vi "Git-Get Repositories.vi"() -> ()   [LabVIEW 2020]
uses:
  Git-Repo JSON Typedef.ctl
  <vilib>/addons/_JKI.lib/REST Client/classes/REST Client/REST Client.lvclass
  <vilib>/JDP Science/JSONtext/JSONtext.lvlib
panel:
  out "Array":T1[](array[typedef])
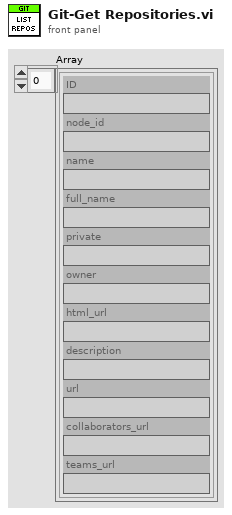
[diagram p1: front panel]
types:
  T1 = typedef "Git-Repo JSON Typedef.ctl" = cluster{"ID":string, "node_id":string, "name":string, "full_name":string, "private":string, "owner":string, "html_url":string, "description":string, "url":string, "collaborators_url":string, "teams_url":string}
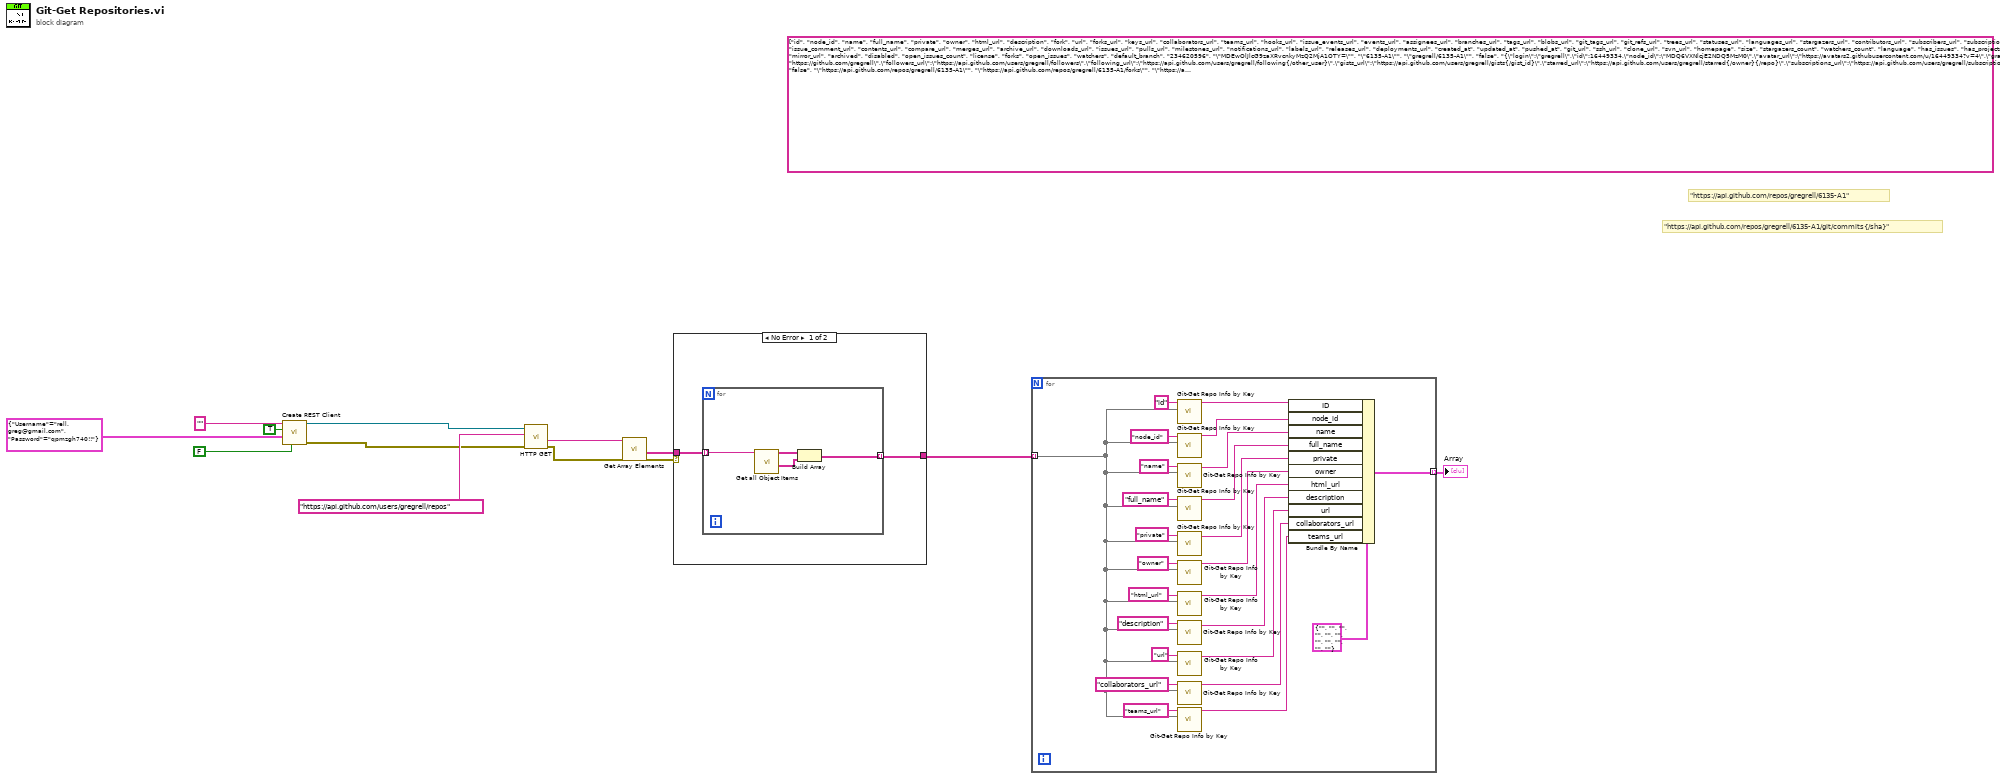
[diagram p0: block diagram]
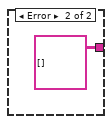
[diagram p2: hidden frame]
diagram:
  (unwired) string[][][] [[["id", "node_id", "name", "full_name", "private", "owner", "html_url", "description", "fork", "url", "forks_url", "keys_url", "collaborators_url", "teams_url", "hooks_url", "issue_events_url", "events_url", "assignees_url", "branches_url", "tags_url", "blobs_url", "git_tags_url", "git_refs_url", "trees_url", "statuses_url", "languages_url", "stargazers_url", "contributors_url", "subscribers_url", "subscription_url", "commits_url", "git_commits_url", "comments_url", "issue_comment_url", "contents_url", "compare_url", "merges_url", "archive_url", "downloads_url", "issues_url", "pulls_url", "milestones_url", "notifications_url", "labels_url", "releases_url", "deployments_url", "created_at", "updated_at", "pushed_at", "git_url", "ssh_url", "clone_url", "svn_url", "homepage", "size", "stargazers_count", "watchers_count", "language", "has_issues", "has_projects", "has_downloads", "has_wiki", "has_pages", "forks_count", "mirror_url", "archived", "disabled", "open_issues_count", "license", "forks", "open_issues", "watchers", "default_branch"], ["234620596", "\"MDEwOlJlcG9zaXRvcnkyMzQ2MjA1OTY=\"", "\"6135-A1\"", "\"gregrell/6135-A1\"", "false", "{\"login\":\"gregrell\",\"id\":16449334,\"node_id\":\"MDQ6VXNlcjE2NDQ5MzM0\",\"avatar_url\":\"https://avatars2.githubusercontent.com/u/16449334?v=4\",\"gravatar_id\":\"\",\"url\":\"https://api.github.com/users/gregrell\",\"html_url\":\"https://github.com/gregrell\",\"followers_url\":\"https://api.github.com/users/gregrell/followers\",\"following_url\":\"https://api.github.com/users/gregrell/following{/other_user}\",\"gists_url\":\"https://api.github.com/users/gregrell/gists{/gist_id}\",\"starred_url\":\"https://api.github.com/users/gregrell/starred{/owner}{/repo}\",\"subscriptions_url\":\"https://api.github.com/users/gregrell/subscriptions\",\"organizations_url\":\"https://api.github.com/users/gregrell/orgs\",\"repos_url\":\"https://api.github.com/users/gregrell/repos\",\"events_url\":\"https://api.github.com/users/gregrell/events{/privacy}\",\"received_events_url\":\"https://api.github.com/users/gregrell/received_events\",\"type\":\"User\",\"site_admin\":false}", "\"https://github.com/gregrell/6135-A1\"", "\"Assignment 1\"", "false", "\"https://api.github.com/repos/gregrell/6135-A1\"", "\"https://api.github.com/repos/gregrell/6135-A1/forks\"", "\"https://api.github.com/repos/gregrell/6135-A1/keys{/key_id}\"", "\"https://api.github.com/repos/gregrell/6135-A1/collaborators{/collaborator}\"", "\"https://api.github.com/repos/gregrell/6135-A1/teams\"", "\"https://api.github.com/repos/gregrell/6135-A1/hooks\"", "\"https://api.github.com/repos/gregrell/6135-A1/issues/events{/number}\"", "\"https://api.github.com/repos/gregrell/6135-A1/events\"", "\"https://api.github.com/repos/gregrell/6135-A1/assignees{/user}\"", "\"https://api.github.com/repos/gregrell/6135-A1/branches{/branch}\"", "\"https://api.github.com/repos/gregrell/6135-A1/tags\"", "\"https://api.github.com/repos/gregrell/6135-A1/git/blobs{/sha}\"", "\"https://api.github.com/repos/gregrell/6135-A1/git/tags{/sha}\"", "\"https://api.github.com/repos/gregrell/6135-A1/git/refs{/sha}\"", "\"https://api.github.com/repos/gregrell/6135-A1/git/trees{/sha}\"", "\"https://api.github.com/repos/gregrell/6135-A1/statuses/{sha}\"", "\"https://api.github.com/repos/gregrell/6135-A1/languages\"", "\"https://api.github.com/repos/gregrell/6135-A1/stargazers\"", "\"https://api.github.com/repos/gregrell/6135-A1/contributors\"", "\"https://api.github.com/repos/gregrell/6135-A1/subscribers\"", "\"https://api.github.com/repos/gregrell/6135-A1/subscription\"", "\"https://api.github.com/repos/gregrell/6135-A1/commits{/sha}\"", "\"https://api.github.com/repos/gregrell/6135-A1/git/commits{/sha}\"", "\"https://api.github.com/repos/gregrell/6135-A1/comments{/number}\"", "\"https://api.github.com/repos/gregrell/6135-A1/issues/comments{/number}\"", "\"https://api.github.com/repos/gregrell/6135-A1/contents/{+path}\"", "\"https://api.github.com/repos/gregrell/6135-A1/compare/{base}...{head}\"", "\"https://api.github.com/repos/gregrell/6135-A1/merges\"", "\"https://api.github.com/repos/gregrell/6135-A1/{archive_format}{/ref}\"", "\"https://api.github.com/repos/gregrell/6135-A1/downloads\"", "\"https://api.github.com/repos/gregrell/6135-A1/issues{/number}\"", "\"https://api.github.com/repos/gregrell/6135-A1/pulls{/number}\"", "\"https://api.github.com/repos/gregrell/6135-A1/milestones{/number}\"", "\"https://api.github.com/repos/gregrell/6135-A1/notifications{?since,all,participating}\"", "\"https://api.github.com/repos/gregrell/6135-A1/labels{/name}\"", "\"https://api.github.com/repos/gregrell/6135-A1/releases{/id}\"", "\"https://api.github.com/repos/gregrell/6135-A1/deployments\"", "\"2020-01-17T19:21:34Z\"", "\"2020-02-04T17:49:57Z\"", "\"2020-02-04T17:49:55Z\"", "\"git://github.com/gregrell/6135-A1.git\"", "\"git@github.com:gregrell/6135-A1.git\"", "\"https://github.com/gregrell/6135-A1.git\"", "\"https://github.com/gregrell/6135-A1\"", "null", "12", "0", "0", "\"C\"", "true", "true", "true", "true", "false", "0", "null", "false", "false", "0", "null", "0", "0", "0", "\"master\""]], [["id", "node_id", "name", "full_name", "private", "owner", "html_url", "description", "fork", "url", "forks_url", "keys_url", "collaborators_url", "teams_url", "hooks_url", "issue_events_url", "events_url", "assignees_url", "branches_url", "tags_url", "blobs_url", "git_tags_url", "git_refs_url", "trees_url", "statuses_url", "languages_url", "stargazers_url", "contributors_url", "subscribers_url", "subscription_url", "commits_url", "git_commits_url", "comments_url", "issue_comment_url", "contents_url", "compare_url", "merges_url", "archive_url", "downloads_url", "issues_url", "pulls_url", "milestones_url", "notifications_url", "labels_url", "releases_url", "deployments_url", "created_at", "updated_at", "pushed_at", "git_url", "ssh_url", "clone_url", "svn_url", "homepage", "size", "stargazers_count", "watchers_count", "language", "has_issues", "has_projects", "has_downloads", "has_wiki", "has_pages", "forks_count", "mirror_url", "archived", "disabled", "open_issues_count", "license", "forks", "open_issues", "watchers", "default_branch"], ["244166740", "\"MDEwOlJlcG9zaXRvcnkyNDQxNjY3NDA=\"", "\"6135-A2\"", "\"gregrell/6135-A2\"", "false", "{\"login\":\"gregrell\",\"id\":16449334,\"node_id\":\"MDQ6VXNlcjE2NDQ5MzM0\",\"avatar_url\":\"https://avatars2.githubusercontent.com/u/16449334?v=4\",\"gravatar_id\":\"\",\"url\":\"https://api.github.com/users/gregrell\",\"html_url\":\"https://github.com/gregrell\",\"followers_url\":\"https://api.github.com/users/gregrell/followers\",\"following_url\":\"https://api.github.com/users/gregrell/following{/other_user}\",\"gists_url\":\"https://api.github.com/users/gregrell/gists{/gist_id}\",\"starred_url\":\"https://api.github.com/users/gregrell/starred{/owner}{/repo}\",\"subscriptions_url\":\"https://api.github.com/users/gregrell/subscriptions\",\"organizations_url\":\"https://api.github.com/users/gregrell/orgs\",\"repos_url\":\"https://api.github.com/users/gregrell/repos\",\"events_url\":\"https://api.github.com/users/gregrell/events{/privacy}\",\"received_events_url\":\"https://api.github.com/users/gregrell/received_events\",\"type\":\"User\",\"site_admin\":false}", "\"https://github.com/gregrell/6135-A2\"", "null", "false", "\"https://api.github.com/repos/gregrell/6135-A2\"", "\"https://api.github.com/repos/gregrell/6135-A2/forks\"", "\"https://api.github.com/repos/gregrell/6135-A2/keys{/key_id}\"", "\"https://api.github.com/repos/gregrell/6135-A2/collaborators{/collaborator}\"", "\"https://api.github.com/repos/gregrell/6135-A2/teams\"", "\"https://api.github.com/repos/gregrell/6135-A2/hooks\"", "\"https://api.github.com/repos/gregrell/6135-A2/issues/events{/number}\"", "\"https://api.github.com/repos/gregrell/6135-A2/events\"", "\"https://api.github.com/repos/gregrell/6135-A2/assignees{/user}\"", "\"https://api.github.com/repos/gregrell/6135-A2/branches{/branch}\"", "\"https://api.github.com/repos/gregrell/6135-A2/tags\"", "\"https://api.github.com/repos/gregrell/6135-A2/git/blobs{/sha}\"", "\"https://api.github.com/repos/gregrell/6135-A2/git/tags{/sha}\"", "\"https://api.github.com/repos/gregrell/6135-A2/git/refs{/sha}\"", "\"https://api.github.com/repos/gregrell/6135-A2/git/trees{/sha}\"", "\"https://api.github.com/repos/gregrell/6135-A2/statuses/{sha}\"", "\"https://api.github.com/repos/gregrell/6135-A2/languages\"", "\"https://api.github.com/repos/gregrell/6135-A2/stargazers\"", "\"https://api.github.com/repos/gregrell/6135-A2/contributors\"", "\"https://api.github.com/repos/gregrell/6135-A2/subscribers\"", "\"https://api.github.com/repos/gregrell/6135-A2/subscription\"", "\"https://api.github.com/repos/gregrell/6135-A2/commits{/sha}\"", "\"https://api.github.com/repos/gregrell/6135-A2/git/commits{/sha}\"", "\"https://api.github.com/repos/gregrell/6135-A2/comments{/number}\"", "\"https://api.github.com/repos/gregrell/6135-A2/issues/comments{/number}\"", "\"https://api.github.com/repos/gregrell/6135-A2/contents/{+path}\"", "\"https://api.github.com/repos/gregrell/6135-A2/compare/{base}...{head}\"", "\"https://api.github.com/repos/gregrell/6135-A2/merges\"", "\"https://api.github.com/repos/gregrell/6135-A2/{archive_format}{/ref}\"", "\"https://api.github.com/repos/gregrell/6135-A2/downloads\"", "\"https://api.github.com/repos/gregrell/6135-A2/issues{/number}\"", "\"https://api.github.com/repos/gregrell/6135-A2/pulls{/number}\"", "\"https://api.github.com/repos/gregrell/6135-A2/milestones{/number}\"", "\"https://api.github.com/repos/gregrell/6135-A2/notifications{?since,all,participating}\"", "\"https://api.github.com/repos/gregrell/6135-A2/labels{/name}\"", "\"https://api.github.com/repos/gregrell/6135-A2/releases{/id}\"", "\"https://api.github.com/repos/gregrell/6135-A2/deployments\"", "\"2020-03-01T14:45:42Z\"", "\"2020-03-03T01:29:14Z\"", "\"2020-03-03T01:29:12Z\"", "\"git://github.com/gregrell/6135-A2.git\"", "\"git@github.com:gregrell/6135-A2.git\"", "\"https://github.com/gregrell/6135-A2.git\"", "\"https://github.com/gregrell/6135-A2\"", "null", "3", "0", "0", "\"Python\"", "true", "true", "true", "true", "false", "0", "null", "false", "false", "1", "null", "0", "1", "0", "\"master\""]], [["id", "node_id", "name", "full_name", "private", "owner", "html_url", "description", "fork", "url", "forks_url", "keys_url", "collaborators_url", "teams_url", "hooks_url", "issue_events_url", "events_url", "assignees_url", "branches_url", "tags_url", "blobs_url", "git_tags_url", "git_refs_url", "trees_url", "statuses_url", "languages_url", "stargazers_url", "contributors_url", "subscribers_url", "subscription_url", "commits_url", "git_commits_url", "comments_url", "issue_comment_url", "contents_url", "compare_url", "merges_url", "archive_url", "downloads_url", "issues_url", "pulls_url", "milestones_url", "notifications_url", "labels_url", "releases_url", "deployments_url", "created_at", "updated_at", "pushed_at", "git_url", "ssh_url", "clone_url", "svn_url", "homepage", "size", "stargazers_count", "watchers_count", "language", "has_issues", "has_projects", "has_downloads", "has_wiki", "has_pages", "forks_count", "mirror_url", "archived", "disabled", "open_issues_count", "license", "forks", "open_issues", "watchers", "default_branch"], ["102971263", "\"MDEwOlJlcG9zaXRvcnkxMDI5NzEyNjM=\"", "\"AIPacMan1\"", "\"gregrell/AIPacMan1\"", "false", "{\"login\":\"gregrell\",\"id\":16449334,\"node_id\":\"MDQ6VXNlcjE2NDQ5MzM0\",\"avatar_url\":\"https://avatars2.githubusercontent.com/u/16449334?v=4\",\"gravatar_id\":\"\",\"url\":\"https://api.github.com/users/gregrell\",\"html_url\":\"https://github.com/gregrell\",\"followers_url\":\"https://api.github.com/users/gregrell/followers\",\"following_url\":\"https://api.github.com/users/gregrell/following{/other_user}\",\"gists_url\":\"https://api.github.com/users/gregrell/gists{/gist_id}\",\"starred_url\":\"https://api.github.com/users/gregrell/starred{/owner}{/repo}\",\"subscriptions_url\":\"https://api.github.com/users/gregrell/subscriptions\",\"organizations_url\":\"https://api.github.com/users/gregrell/orgs\",\"repos_url\":\"https://api.github.com/users/gregrell/repos\",\"events_url\":\"https://api.github.com/users/gregrell/events{/privacy}\",\"received_events_url\":\"https://api.github.com/users/gregrell/received_events\",\"type\":\"User\",\"site_admin\":false}", "\"https://github.com/gregrell/AIPacMan1\"", "\"AI Class Pacman assignment 1\"", "false", "\"https://api.github.com/repos/gregrell/AIPacMan1\"", "\"https://api.github.com/repos/gregrell/AIPacMan1/forks\"", "\"https://api.github.com/repos/gregrell/AIPacMan1/keys{/key_id}\"", "\"https://api.github.com/repos/gregrell/AIPacMan1/collaborators{/collaborator}\"", "\"https://api.github.com/repos/gregrell/AIPacMan1/teams\"", "\"https://api.github.com/repos/gregrell/AIPacMan1/hooks\"", "\"https://api.github.com/repos/gregrell/AIPacMan1/issues/events{/number}\"", "\"https://api.github.com/repos/gregrell/AIPacMan1/events\"", "\"https://api.github.com/repos/gregrell/AIPacMan1/assignees{/user}\"", "\"https://api.github.com/repos/gregrell/AIPacMan1/branches{/branch}\"", "\"https://api.github.com/repos/gregrell/AIPacMan1/tags\"", "\"https://api.github.com/repos/gregrell/AIPacMan1/git/blobs{/sha}\"", "\"https://api.github.com/repos/gregrell/AIPacMan1/git/tags{/sha}\"", "\"https://api.github.com/repos/gregrell/AIPacMan1/git/refs{/sha}\"", "\"https://api.github.com/repos/gregrell/AIPacMan1/git/trees{/sha}\"", "\"https://api.github.com/repos/gregrell/AIPacMan1/statuses/{sha}\"", "\"https://api.github.com/repos/gregrell/AIPacMan1/languages\"", "\"https://api.github.com/repos/gregrell/AIPacMan1/stargazers\"", "\"https://api.github.com/repos/gregrell/AIPacMan1/contributors\"", "\"https://api.github.com/repos/gregrell/AIPacMan1/subscribers\"", "\"https://api.github.com/repos/gregrell/AIPacMan1/subscription\"", "\"https://api.github.com/repos/gregrell/AIPacMan1/commits{/sha}\"", "\"https://api.github.com/repos/gregrell/AIPacMan1/git/commits{/sha}\"", "\"https://api.github.com/repos/gregrell/AIPacMan1/comments{/number}\"", "\"https://api.github.com/repos/gregrell/AIPacMan1/issues/comments{/number}\"", "\"https://api.github.com/repos/gregrell/AIPacMan1/contents/{+path}\"", "\"https://api.github.com/repos/gregrell/AIPacMan1/compare/{base}...{head}\"", "\"https://api.github.com/repos/gregrell/AIPacMan1/merges\"", "\"https://api.github.com/repos/gregrell/AIPacMan1/{archive_format}{/ref}\"", "\"https://api.github.com/repos/gregrell/AIPacMan1/downloads\"", "\"https://api.github.com/repos/gregrell/AIPacMan1/issues{/number}\"", "\"https://api.github.com/repos/gregrell/AIPacMan1/pulls{/number}\"", "\"https://api.github.com/repos/gregrell/AIPacMan1/milestones{/number}\"", "\"https://api.github.com/repos/gregrell/AIPacMan1/notifications{?since,all,participating}\"", "\"https://api.github.com/repos/gregrell/AIPacMan1/labels{/name}\"", "\"https://api.github.com/repos/gregrell/AIPacMan1/releases{/id}\"", "\"https://api.github.com/repos/gregrell/AIPacMan1/deployments\"", "\"2017-09-09T17:04:38Z\"", "\"2017-09-09T17:06:54Z\"", "\"2017-10-05T17:59:55Z\"", "\"git://github.com/gregrell/AIPacMan1.git\"", "\"git@github.com:gregrell/AIPacMan1.git\"", "\"https://github.com/gregrell/AIPacMan1.git\"", "\"https://github.com/gregrell/AIPacMan1\"", "null", "277", "0", "0", "\"Python\"", "true", "true", "true", "true", "false", "0", "null", "false", "false", "0", "null", "0", "0", "0", "\"master\""]], [["id", "node_id", "name", "full_name", "private", "owner", "html_url", "description", "fork", "url", "forks_url", "keys_url", "collaborators_url", "teams_url", "hooks_url", "issue_events_url", "events_url", "assignees_url", "branches_url", "tags_url", "blobs_url", "git_tags_url", "git_refs_url", "trees_url", "statuses_url", "languages_url", "stargazers_url", "contributors_url", "subscribers_url", "subscription_url", "commits_url", "git_commits_url", "comments_url", "issue_comment_url", "contents_url", "compare_url", "merges_url", "archive_url", "downloads_url", "issues_url", "pulls_url", "milestones_url", "notifications_url", "labels_url", "releases_url", "deployments_url", "created_at", "updated_at", "pushed_at", "git_url", "ssh_url", "clone_url", "svn_url", "homepage", "size", "stargazers_count", "watchers_count", "language", "has_issues", "has_projects", "has_downloads", "has_wiki", "has_pages", "forks_count", "mirror_url", "archived", "disabled", "open_issues_count", "license", "forks", "open_issues", "watchers", "default_branch"], ["108994983", "\"MDEwOlJlcG9zaXRvcnkxMDg5OTQ5ODM=\"", "\"AIPacMan2\"", "\"gregrell/AIPacMan2\"", "false", "{\"login\":\"gregrell\",\"id\":16449334,\"node_id\":\"MDQ6VXNlcjE2NDQ5MzM0\",\"avatar_url\":\"https://avatars2.githubusercontent.com/u/16449334?v=4\",\"gravatar_id\":\"\",\"url\":\"https://api.github.com/users/gregrell\",\"html_url\":\"https://github.com/gregrell\",\"followers_url\":\"https://api.github.com/users/gregrell/followers\",\"following_url\":\"https://api.github.com/users/gregrell/following{/other_user}\",\"gists_url\":\"https://api.github.com/users/gregrell/gists{/gist_id}\",\"starred_url\":\"https://api.github.com/users/gregrell/starred{/owner}{/repo}\",\"subscriptions_url\":\"https://api.github.com/users/gregrell/subscriptions\",\"organizations_url\":\"https://api.github.com/users/gregrell/orgs\",\"repos_url\":\"https://api.github.com/users/gregrell/repos\",\"events_url\":\"https://api.github.com/users/gregrell/events{/privacy}\",\"received_events_url\":\"https://api.github.com/users/gregrell/received_events\",\"type\":\"User\",\"site_admin\":false}", "\"https://github.com/gregrell/AIPacMan2\"", "\"Berkley AI course project 3\"", "false", "\"https://api.github.com/repos/gregrell/AIPacMan2\"", "\"https://api.github.com/repos/gregrell/AIPacMan2/forks\"", "\"https://api.github.com/repos/gregrell/AIPacMan2/keys{/key_id}\"", "\"https://api.github.com/repos/gregrell/AIPacMan2/collaborators{/collaborator}\"", "\"https://api.github.com/repos/gregrell/AIPacMan2/teams\"", "\"https://api.github.com/repos/gregrell/AIPacMan2/hooks\"", "\"https://api.github.com/repos/gregrell/AIPacMan2/issues/events{/number}\"", "\"https://api.github.com/repos/gregrell/AIPacMan2/events\"", "\"https://api.github.com/repos/gregrell/AIPacMan2/assignees{/user}\"", "\"https://api.github.com/repos/gregrell/AIPacMan2/branches{/branch}\"", "\"https://api.github.com/repos/gregrell/AIPacMan2/tags\"", "\"https://api.github.com/repos/gregrell/AIPacMan2/git/blobs{/sha}\"", "\"https://api.github.com/repos/gregrell/AIPacMan2/git/tags{/sha}\"", "\"https://api.github.com/repos/gregrell/AIPacMan2/git/refs{/sha}\"", "\"https://api.github.com/repos/gregrell/AIPacMan2/git/trees{/sha}\"", "\"https://api.github.com/repos/gregrell/AIPacMan2/statuses/{sha}\"", "\"https://api.github.com/repos/gregrell/AIPacMan2/languages\"", "\"https://api.github.com/repos/gregrell/AIPacMan2/stargazers\"", "\"https://api.github.com/repos/gregrell/AIPacMan2/contributors\"", "\"https://api.github.com/repos/gregrell/AIPacMan2/subscribers\"", "\"https://api.github.com/repos/gregrell/AIPacMan2/subscription\"", "\"https://api.github.com/repos/gregrell/AIPacMan2/commits{/sha}\"", "\"https://api.github.com/repos/gregrell/AIPacMan2/git/commits{/sha}\"", "\"https://api.github.com/repos/gregrell/AIPacMan2/comments{/number}\"", "\"https://api.github.com/repos/gregrell/AIPacMan2/issues/comments{/number}\"", "\"https://api.github.com/repos/gregrell/AIPacMan2/contents/{+path}\"", "\"https://api.github.com/repos/gregrell/AIPacMan2/compare/{base}...{head}\"", "\"https://api.github.com/repos/gregrell/AIPacMan2/merges\"", "\"https://api.github.com/repos/gregrell/AIPacMan2/{archive_format}{/ref}\"", "\"https://api.github.com/repos/gregrell/AIPacMan2/downloads\"", "\"https://api.github.com/repos/gregrell/AIPacMan2/issues{/number}\"", "\"https://api.github.com/repos/gregrell/AIPacMan2/pulls{/number}\"", "\"https://api.github.com/repos/gregrell/AIPacMan2/milestones{/number}\"", "\"https://api.github.com/repos/gregrell/AIPacMan2/notifications{?since,all,participating}\"", "\"https://api.github.com/repos/gregrell/AIPacMan2/labels{/name}\"", "\"https://api.github.com/repos/gregrell/AIPacMan2/releases{/id}\"", "\"https://api.github.com/repos/gregrell/AIPacMan2/deployments\"", "\"2017-10-31T12:50:33Z\"", "\"2017-10-31T12:54:09Z\"", "\"2017-11-19T15:26:08Z\"", "\"git://github.com/gregrell/AIPacMan2.git\"", "\"git@github.com:gregrell/AIPacMan2.git\"", "\"https://github.com/gregrell/AIPacMan2.git\"", "\"https://github.com/gregrell/AIPacMan2\"", "null", "421", "0", "0", "\"Python\"", "true", "true", "true", "true", "false", "0", "null", "false", "false", "0", "null", "0", "0", "0", "\"master\""]], [["id", "node_id", "name", "full_name", "private", "owner", "html_url", "description", "fork", "url", "forks_url", "keys_url", "collaborators_url", "teams_url", "hooks_url", "issue_events_url", "events_url", "assignees_url", "branches_url", "tags_url", "blobs_url", "git_tags_url", "git_refs_url", "trees_url", "statuses_url", "languages_url", "stargazers_url", "contributors_url", "subscribers_url", "subscription_url", "commits_url", "git_commits_url", "comments_url", "issue_comment_url", "contents_url", "compare_url", "merges_url", "archive_url", "downloads_url", "issues_url", "pulls_url", "milestones_url", "notifications_url", "labels_url", "releases_url", "deployments_url", "created_at", "updated_at", "pushed_at", "git_url", "ssh_url", "clone_url", "svn_url", "homepage", "size", "stargazers_count", "watchers_count", "language", "has_issues", "has_projects", "has_downloads", "has_wiki", "has_pages", "forks_count", "mirror_url", "archived", "disabled", "open_issues_count", "license", "forks", "open_issues", "watchers", "default_branch"], ["108542536", "\"MDEwOlJlcG9zaXRvcnkxMDg1NDI1MzY=\"", "\"CNT5008NetworkSim\"", "\"gregrell/CNT5008NetworkSim\"", "false", "{\"login\":\"gregrell\",\"id\":16449334,\"node_id\":\"MDQ6VXNlcjE2NDQ5MzM0\",\"avatar_url\":\"https://avatars2.githubusercontent.com/u/16449334?v=4\",\"gravatar_id\":\"\",\"url\":\"https://api.github.com/users/gregrell\",\"html_url\":\"https://github.com/gregrell\",\"followers_url\":\"https://api.github.com/users/gregrell/followers\",\"following_url\":\"https://api.github.com/users/gregrell/following{/other_user}\",\"gists_url\":\"https://api.github.com/users/gregrell/gists{/gist_id}\",\"starred_url\":\"https://api.github.com/users/gregrell/starred{/owner}{/repo}\",\"subscriptions_url\":\"https://api.github.com/users/gregrell/subscriptions\",\"organizations_url\":\"https://api.github.com/users/gregrell/orgs\",\"repos_url\":\"https://api.github.com/users/gregrell/repos\",\"events_url\":\"https://api.github.com/users/gregrell/events{/privacy}\",\"received_events_url\":\"https://api.github.com/users/gregrell/received_events\",\"type\":\"User\",\"site_admin\":false}", "\"https://github.com/gregrell/CNT5008NetworkSim\"", "\"CNT5008 Programming Assignment\"", "false", "\"https://api.github.com/repos/gregrell/CNT5008NetworkSim\"", "\"https://api.github.com/repos/gregrell/CNT5008NetworkSim/forks\"", "\"https://api.github.com/repos/gregrell/CNT5008NetworkSim/keys{/key_id}\"", "\"https://api.github.com/repos/gregrell/CNT5008NetworkSim/collaborators{/collaborator}\"", "\"https://api.github.com/repos/gregrell/CNT5008NetworkSim/teams\"", "\"https://api.github.com/repos/gregrell/CNT5008NetworkSim/hooks\"", "\"https://api.github.com/repos/gregrell/CNT5008NetworkSim/issues/events{/number}\"", "\"https://api.github.com/repos/gregrell/CNT5008NetworkSim/events\"", "\"https://api.github.com/repos/gregrell/CNT5008NetworkSim/assignees{/user}\"", "\"https://api.github.com/repos/gregrell/CNT5008NetworkSim/branches{/branch}\"", "\"https://api.github.com/repos/gregrell/CNT5008NetworkSim/tags\"", "\"https://api.github.com/repos/gregrell/CNT5008NetworkSim/git/blobs{/sha}\"", "\"https://api.github.com/repos/gregrell/CNT5008NetworkSim/git/tags{/sha}\"", "\"https://api.github.com/repos/gregrell/CNT5008NetworkSim/git/refs{/sha}\"", "\"https://api.github.com/repos/gregrell/CNT5008NetworkSim/git/trees{/sha}\"", "\"https://api.github.com/repos/gregrell/CNT5008NetworkSim/statuses/{sha}\"", "\"https://api.github.com/repos/gregrell/CNT5008NetworkSim/languages\"", "\"https://api.github.com/repos/gregrell/CNT5008NetworkSim/stargazers\"", "\"https://api.github.com/repos/gregrell/CNT5008NetworkSim/contributors\"", "\"https://api.github.com/repos/gregrell/CNT5008NetworkSim/subscribers\"", "\"https://api.github.com/repos/gregrell/CNT5008NetworkSim/subscription\"", "\"https://api.github.com/repos/gregrell/CNT5008NetworkSim/commits{/sha}\"", "\"https://api.github.com/repos/gregrell/CNT5008NetworkSim/git/commits{/sha}\"", "\"https://api.github.com/repos/gregrell/CNT5008NetworkSim/comments{/number}\"", "\"https://api.github.com/repos/gregrell/CNT5008NetworkSim/issues/comments{/number}\"", "\"https://api.github.com/repos/gregrell/CNT5008NetworkSim/contents/{+path}\"", "\"https://api.github.com/repos/gregrell/CNT5008NetworkSim/compare/{base}...{head}\"", "\"https://api.github.com/repos/gregrell/CNT5008NetworkSim/merges\"", "\"https://api.github.com/repos/gregrell/CNT5008NetworkSim/{archive_format}{/ref}\"", "\"https://api.github.com/repos/gregrell/CNT5008NetworkSim/downloads\"", "\"https://api.github.com/repos/gregrell/CNT5008NetworkSim/issues{/number}\"", "\"https://api.github.com/repos/gregrell/CNT5008NetworkSim/pulls{/number}\"", "\"https://api.github.com/repos/gregrell/CNT5008NetworkSim/milestones{/number}\"", "\"https://api.github.com/repos/gregrell/CNT5008NetworkSim/notifications{?since,all,participating}\"", "\"https://api.github.com/repos/gregrell/CNT5008NetworkSim/labels{/name}\"", "\"https://api.github.com/repos/gregrell/CNT5008NetworkSim/releases{/id}\"", "\"https://api.github.com/repos/gregrell/CNT5008NetworkSim/deployments\"", "\"2017-10-27T12:19:49Z\"", "\"2017-10-27T12:21:19Z\"", "\"2017-11-27T02:09:06Z\"", "\"git://github.com/gregrell/CNT5008NetworkSim.git\"", "\"git@github.com:gregrell/CNT5008NetworkSim.git\"", "\"https://github.com/gregrell/CNT5008NetworkSim.git\"", "\"https://github.com/gregrell/CNT5008NetworkSim\"", "null", "258", "0", "0", "\"HTML\"", "true", "true", "true", "true", "false", "0", "null", "false", "false", "0", "null", "0", "0", "0", "\"master\""]], [["id", "node_id", "name", "full_name", "private", "owner", "html_url", "description", "fork", "url", "forks_url", "keys_url", "collaborators_url", "teams_url", "hooks_url", "issue_events_url", "events_url", "assignees_url", "branches_url", "tags_url", "blobs_url", "git_tags_url", "git_refs_url", "trees_url", "statuses_url", "languages_url", "stargazers_url", "contributors_url", "subscribers_url", "subscription_url", "commits_url", "git_commits_url", "comments_url", "issue_comment_url", "contents_url", "compare_url", "merges_url", "archive_url", "downloads_url", "issues_url", "pulls_url", "milestones_url", "notifications_url", "labels_url", "releases_url", "deployments_url", "created_at", "updated_at", "pushed_at", "git_url", "ssh_url", "clone_url", "svn_url", "homepage", "size", "stargazers_count", "watchers_count", "language", "has_issues", "has_projects", "has_downloads", "has_wiki", "has_pages", "forks_count", "mirror_url", "archived", "disabled", "open_issues_count", "license", "forks", "open_issues", "watchers", "default_branch"], ["263786389", "\"MDEwOlJlcG9zaXRvcnkyNjM3ODYzODk=\"", "\"consoleApp\"", "\"gregrell/consoleApp\"", "false", "{\"login\":\"gregrell\",\"id\":16449334,\"node_id\":\"MDQ6VXNlcjE2NDQ5MzM0\",\"avatar_url\":\"https://avatars2.githubusercontent.com/u/16449334?v=4\",\"gravatar_id\":\"\",\"url\":\"https://api.github.com/users/gregrell\",\"html_url\":\"https://github.com/gregrell\",\"followers_url\":\"https://api.github.com/users/gregrell/followers\",\"following_url\":\"https://api.github.com/users/gregrell/following{/other_user}\",\"gists_url\":\"https://api.github.com/users/gregrell/gists{/gist_id}\",\"starred_url\":\"https://api.github.com/users/gregrell/starred{/owner}{/repo}\",\"subscriptions_url\":\"https://api.github.com/users/gregrell/subscriptions\",\"organizations_url\":\"https://api.github.com/users/gregrell/orgs\",\"repos_url\":\"https://api.github.com/users/gregrell/repos\",\"events_url\":\"https://api.github.com/users/gregrell/events{/privacy}\",\"received_events_url\":\"https://api.github.com/users/gregrell/received_events\",\"type\":\"User\",\"site_admin\":false}", "\"https://github.com/gregrell/consoleApp\"", "null", "false", "\"https://api.github.com/repos/gregrell/consoleApp\"", "\"https://api.github.com/repos/gregrell/consoleApp/forks\"", "\"https://api.github.com/repos/gregrell/consoleApp/keys{/key_id}\"", "\"https://api.github.com/repos/gregrell/consoleApp/collaborators{/collaborator}\"", "\"https://api.github.com/repos/gregrell/consoleApp/teams\"", "\"https://api.github.com/repos/gregrell/consoleApp/hooks\"", "\"https://api.github.com/repos/gregrell/consoleApp/issues/events{/number}\"", "\"https://api.github.com/repos/gregrell/consoleApp/events\"", "\"https://api.github.com/repos/gregrell/consoleApp/assignees{/user}\"", "\"https://api.github.com/repos/gregrell/consoleApp/branches{/branch}\"", "\"https://api.github.com/repos/gregrell/consoleApp/tags\"", "\"https://api.github.com/repos/gregrell/consoleApp/git/blobs{/sha}\"", "\"https://api.github.com/repos/gregrell/consoleApp/git/tags{/sha}\"", "\"https://api.github.com/repos/gregrell/consoleApp/git/refs{/sha}\"", "\"https://api.github.com/repos/gregrell/consoleApp/git/trees{/sha}\"", "\"https://api.github.com/repos/gregrell/consoleApp/statuses/{sha}\"", "\"https://api.github.com/repos/gregrell/consoleApp/languages\"", "\"https://api.github.com/repos/gregrell/consoleApp/stargazers\"", "\"https://api.github.com/repos/gregrell/consoleApp/contributors\"", "\"https://api.github.com/repos/gregrell/consoleApp/subscribers\"", "\"https://api.github.com/repos/gregrell/consoleApp/subscription\"", "\"https://api.github.com/repos/gregrell/consoleApp/commits{/sha}\"", "\"https://api.github.com/repos/gregrell/consoleApp/git/commits{/sha}\"", "\"https://api.github.com/repos/gregrell/consoleApp/comments{/number}\"", "\"https://api.github.com/repos/gregrell/consoleApp/issues/comments{/number}\"", "\"https://api.github.com/repos/gregrell/consoleApp/contents/{+path}\"", "\"https://api.github.com/repos/gregrell/consoleApp/compare/{base}...{head}\"", "\"https://api.github.com/repos/gregrell/consoleApp/merges\"", "\"https://api.github.com/repos/gregrell/consoleApp/{archive_format}{/ref}\"", "\"https://api.github.com/repos/gregrell/consoleApp/downloads\"", "\"https://api.github.com/repos/gregrell/consoleApp/issues{/number}\"", "\"https://api.github.com/repos/gregrell/consoleApp/pulls{/number}\"", "\"https://api.github.com/repos/gregrell/consoleApp/milestones{/number}\"", "\"https://api.github.com/repos/gregrell/consoleApp/notifications{?since,all,participating}\"", "\"https://api.github.com/repos/gregrell/consoleApp/labels{/name}\"", "\"https://api.github.com/repos/gregrell/consoleApp/releases{/id}\"", "\"https://api.github.com/repos/gregrell/consoleApp/deployments\"", "\"2020-05-14T01:39:34Z\"", "\"2020-05-14T01:39:34Z\"", "\"2020-05-14T01:39:35Z\"", "\"git://github.com/gregrell/consoleApp.git\"", "\"git@github.com:gregrell/consoleApp.git\"", "\"https://github.com/gregrell/consoleApp.git\"", "\"https://github.com/gregrell/consoleApp\"", "null", "0", "0", "0", "null", "true", "true", "true", "true", "false", "0", "null", "false", "false", "0", "null", "0", "0", "0", "\"master\""]], [["id", "node_id", "name", "full_name", "private", "owner", "html_url", "description", "fork", "url", "forks_url", "keys_url", "collaborators_url", "teams_url", "hooks_url", "issue_events_url", "events_url", "assignees_url", "branches_url", "tags_url", "blobs_url", "git_tags_url", "git_refs_url", "trees_url", "statuses_url", "languages_url", "stargazers_url", "contributors_url", "subscribers_url", "subscription_url", "commits_url", "git_commits_url", "comments_url", "issue_comment_url", "contents_url", "compare_url", "merges_url", "archive_url", "downloads_url", "issues_url", "pulls_url", "milestones_url", "notifications_url", "labels_url", "releases_url", "deployments_url", "created_at", "updated_at", "pushed_at", "git_url", "ssh_url", "clone_url", "svn_url", "homepage", "size", "stargazers_count", "watchers_count", "language", "has_issues", "has_projects", "has_downloads", "has_wiki", "has_pages", "forks_count", "mirror_url", "archived", "disabled", "open_issues_count", "license", "forks", "open_issues", "watchers", "default_branch"], ["71506781", "\"MDEwOlJlcG9zaXRvcnk3MTUwNjc4MQ==\"", "\"COT_Project\"", "\"gregrell/COT_Project\"", "false", "{\"login\":\"gregrell\",\"id\":16449334,\"node_id\":\"MDQ6VXNlcjE2NDQ5MzM0\",\"avatar_url\":\"https://avatars2.githubusercontent.com/u/16449334?v=4\",\"gravatar_id\":\"\",\"url\":\"https://api.github.com/users/gregrell\",\"html_url\":\"https://github.com/gregrell\",\"followers_url\":\"https://api.github.com/users/gregrell/followers\",\"following_url\":\"https://api.github.com/users/gregrell/following{/other_user}\",\"gists_url\":\"https://api.github.com/users/gregrell/gists{/gist_id}\",\"starred_url\":\"https://api.github.com/users/gregrell/starred{/owner}{/repo}\",\"subscriptions_url\":\"https://api.github.com/users/gregrell/subscriptions\",\"organizations_url\":\"https://api.github.com/users/gregrell/orgs\",\"repos_url\":\"https://api.github.com/users/gregrell/repos\",\"events_url\":\"https://api.github.com/users/gregrell/events{/privacy}\",\"received_events_url\":\"https://api.github.com/users/gregrell/received_events\",\"type\":\"User\",\"site_admin\":false}", "\"https://github.com/gregrell/COT_Project\"", "\"COT class design project\"", "false", "\"https://api.github.com/repos/gregrell/COT_Project\"", "\"https://api.github.com/repos/gregrell/COT_Project/forks\"", "\"https://api.github.com/repos/gregrell/COT_Project/keys{/key_id}\"", "\"https://api.github.com/repos/gregrell/COT_Project/collaborators{/collaborator}\"", "\"https://api.github.com/repos/gregrell/COT_Project/teams\"", "\"https://api.github.com/repos/gregrell/COT_Project/hooks\"", "\"https://api.github.com/repos/gregrell/COT_Project/issues/events{/number}\"", "\"https://api.github.com/repos/gregrell/COT_Project/events\"", "\"https://api.github.com/repos/gregrell/COT_Project/assignees{/user}\"", "\"https://api.github.com/repos/gregrell/COT_Project/branches{/branch}\"", "\"https://api.github.com/repos/gregrell/COT_Project/tags\"", "\"https://api.github.com/repos/gregrell/COT_Project/git/blobs{/sha}\"", "\"https://api.github.com/repos/gregrell/COT_Project/git/tags{/sha}\"", "\"https://api.github.com/repos/gregrell/COT_Project/git/refs{/sha}\"", "\"https://api.github.com/repos/gregrell/COT_Project/git/trees{/sha}\"", "\"https://api.github.com/repos/gregrell/COT_Project/statuses/{sha}\"", "\"https://api.github.com/repos/gregrell/COT_Project/languages\"", "\"https://api.github.com/repos/gregrell/COT_Project/stargazers\"", "\"https://api.github.com/repos/gregrell/COT_Project/contributors\"", "\"https://api.github.com/repos/gregrell/COT_Project/subscribers\"", "\"https://api.github.com/repos/gregrell/COT_Project/subscription\"", "\"https://api.github.com/repos/gregrell/COT_Project/commits{/sha}\"", "\"https://api.github.com/repos/gregrell/COT_Project/git/commits{/sha}\"", "\"https://api.github.com/repos/gregrell/COT_Project/comments{/number}\"", "\"https://api.github.com/repos/gregrell/COT_Project/issues/comments{/number}\"", "\"https://api.github.com/repos/gregrell/COT_Project/contents/{+path}\"", "\"https://api.github.com/repos/gregrell/COT_Project/compare/{base}...{head}\"", "\"https://api.github.com/repos/gregrell/COT_Project/merges\"", "\"https://api.github.com/repos/gregrell/COT_Project/{archive_format}{/ref}\"", "\"https://api.github.com/repos/gregrell/COT_Project/downloads\"", "\"https://api.github.com/repos/gregrell/COT_Project/issues{/number}\"", "\"https://api.github.com/repos/gregrell/COT_Project/pulls{/number}\"", "\"https://api.github.com/repos/gregrell/COT_Project/milestones{/number}\"", "\"https://api.github.com/repos/gregrell/COT_Project/notifications{?since,all,participating}\"", "\"https://api.github.com/repos/gregrell/COT_Project/labels{/name}\"", "\"https://api.github.com/repos/gregrell/COT_Project/releases{/id}\"", "\"https://api.github.com/repos/gregrell/COT_Project/deployments\"", "\"2016-10-20T21:43:17Z\"", "\"2016-10-20T21:58:00Z\"", "\"2016-12-10T22:06:32Z\"", "\"git://github.com/gregrell/COT_Project.git\"", "\"git@github.com:gregrell/COT_Project.git\"", "\"https://github.com/gregrell/COT_Project.git\"", "\"https://github.com/gregrell/COT_Project\"", "null", "158", "0", "0", "\"Java\"", "true", "true", "true", "true", "false", "1", "null", "false", "false", "0", "null", "1", "0", "0", "\"master\""]], [["id", "node_id", "name", "full_name", "private", "owner", "html_url", "description", "fork", "url", "forks_url", "keys_url", "collaborators_url", "teams_url", "hooks_url", "issue_events_url", "events_url", "assignees_url", "branches_url", "tags_url", "blobs_url", "git_tags_url", "git_refs_url", "trees_url", "statuses_url", "languages_url", "stargazers_url", "contributors_url", "subscribers_url", "subscription_url", "commits_url", "git_commits_url", "comments_url", "issue_comment_url", "contents_url", "compare_url", "merges_url", "archive_url", "downloads_url", "issues_url", "pulls_url", "milestones_url", "notifications_url", "labels_url", "releases_url", "deployments_url", "created_at", "updated_at", "pushed_at", "git_url", "ssh_url", "clone_url", "svn_url", "homepage", "size", "stargazers_count", "watchers_count", "language", "has_issues", "has_projects", "has_downloads", "has_wiki", "has_pages", "forks_count", "mirror_url", "archived", "disabled", "open_issues_count", "license", "forks", "open_issues", "watchers", "default_branch"], ["220771396", "\"MDEwOlJlcG9zaXRvcnkyMjA3NzEzOTY=\"", "\"FinalProject\"", "\"gregrell/FinalProject\"", "false", "{\"login\":\"gregrell\",\"id\":16449334,\"node_id\":\"MDQ6VXNlcjE2NDQ5MzM0\",\"avatar_url\":\"https://avatars2.githubusercontent.com/u/16449334?v=4\",\"gravatar_id\":\"\",\"url\":\"https://api.github.com/users/gregrell\",\"html_url\":\"https://github.com/gregrell\",\"followers_url\":\"https://api.github.com/users/gregrell/followers\",\"following_url\":\"https://api.github.com/users/gregrell/following{/other_user}\",\"gists_url\":\"https://api.github.com/users/gregrell/gists{/gist_id}\",\"starred_url\":\"https://api.github.com/users/gregrell/starred{/owner}{/repo}\",\"subscriptions_url\":\"https://api.github.com/users/gregrell/subscriptions\",\"organizations_url\":\"https://api.github.com/users/gregrell/orgs\",\"repos_url\":\"https://api.github.com/users/gregrell/repos\",\"events_url\":\"https://api.github.com/users/gregrell/events{/privacy}\",\"received_events_url\":\"https://api.github.com/users/gregrell/received_events\",\"type\":\"User\",\"site_admin\":false}", "\"https://github.com/gregrell/FinalProject\"", "\"Advanced Text Mining Final Project\"", "false", "\"https://api.github.com/repos/gregrell/FinalProject\"", "\"https://api.github.com/repos/gregrell/FinalProject/forks\"", "\"https://api.github.com/repos/gregrell/FinalProject/keys{/key_id}\"", "\"https://api.github.com/repos/gregrell/FinalProject/collaborators{/collaborator}\"", "\"https://api.github.com/repos/gregrell/FinalProject/teams\"", "\"https://api.github.com/repos/gregrell/FinalProject/hooks\"", "\"https://api.github.com/repos/gregrell/FinalProject/issues/events{/number}\"", "\"https://api.github.com/repos/gregrell/FinalProject/events\"", "\"https://api.github.com/repos/gregrell/FinalProject/assignees{/user}\"", "\"https://api.github.com/repos/gregrell/FinalProject/branches{/branch}\"", "\"https://api.github.com/repos/gregrell/FinalProject/tags\"", "\"https://api.github.com/repos/gregrell/FinalProject/git/blobs{/sha}\"", "\"https://api.github.com/repos/gregrell/FinalProject/git/tags{/sha}\"", "\"https://api.github.com/repos/gregrell/FinalProject/git/refs{/sha}\"", "\"https://api.github.com/repos/gregrell/FinalProject/git/trees{/sha}\"", "\"https://api.github.com/repos/gregrell/FinalProject/statuses/{sha}\"", "\"https://api.github.com/repos/gregrell/FinalProject/languages\"", "\"https://api.github.com/repos/gregrell/FinalProject/stargazers\"", "\"https://api.github.com/repos/gregrell/FinalProject/contributors\"", "\"https://api.github.com/repos/gregrell/FinalProject/subscribers\"", "\"https://api.github.com/repos/gregrell/FinalProject/subscription\"", "\"https://api.github.com/repos/gregrell/FinalProject/commits{/sha}\"", "\"https://api.github.com/repos/gregrell/FinalProject/git/commits{/sha}\"", "\"https://api.github.com/repos/gregrell/FinalProject/comments{/number}\"", "\"https://api.github.com/repos/gregrell/FinalProject/issues/comments{/number}\"", "\"https://api.github.com/repos/gregrell/FinalProject/contents/{+path}\"", "\"https://api.github.com/repos/gregrell/FinalProject/compare/{base}...{head}\"", "\"https://api.github.com/repos/gregrell/FinalProject/merges\"", "\"https://api.github.com/repos/gregrell/FinalProject/{archive_format}{/ref}\"", "\"https://api.github.com/repos/gregrell/FinalProject/downloads\"", "\"https://api.github.com/repos/gregrell/FinalProject/issues{/number}\"", "\"https://api.github.com/repos/gregrell/FinalProject/pulls{/number}\"", "\"https://api.github.com/repos/gregrell/FinalProject/milestones{/number}\"", "\"https://api.github.com/repos/gregrell/FinalProject/notifications{?since,all,participating}\"", "\"https://api.github.com/repos/gregrell/FinalProject/labels{/name}\"", "\"https://api.github.com/repos/gregrell/FinalProject/releases{/id}\"", "\"https://api.github.com/repos/gregrell/FinalProject/deployments\"", "\"2019-11-10T10:01:13Z\"", "\"2019-12-11T03:21:52Z\"", "\"2019-12-11T03:21:50Z\"", "\"git://github.com/gregrell/FinalProject.git\"", "\"git@github.com:gregrell/FinalProject.git\"", "\"https://github.com/gregrell/FinalProject.git\"", "\"https://github.com/gregrell/FinalProject\"", "null", "302", "0", "0", "\"Python\"", "true", "true", "true", "true", "false", "0", "null", "false", "false", "0", "null", "0", "0", "0", "\"master\""]], [["id", "node_id", "name", "full_name", "private", "owner", "html_url", "description", "fork", "url", "forks_url", "keys_url", "collaborators_url", "teams_url", "hooks_url", "issue_events_url", "events_url", "assignees_url", "branches_url", "tags_url", "blobs_url", "git_tags_url", "git_refs_url", "trees_url", "statuses_url", "languages_url", "stargazers_url", "contributors_url", "subscribers_url", "subscription_url", "commits_url", "git_commits_url", "comments_url", "issue_comment_url", "contents_url", "compare_url", "merges_url", "archive_url", "downloads_url", "issues_url", "pulls_url", "milestones_url", "notifications_url", "labels_url", "releases_url", "deployments_url", "created_at", "updated_at", "pushed_at", "git_url", "ssh_url", "clone_url", "svn_url", "homepage", "size", "stargazers_count", "watchers_count", "language", "has_issues", "has_projects", "has_downloads", "has_wiki", "has_pages", "forks_count", "mirror_url", "archived", "disabled", "open_issues_count", "license", "forks", "open_issues", "watchers", "default_branch"], ["208271047", "\"MDEwOlJlcG9zaXRvcnkyMDgyNzEwNDc=\"", "\"HW1\"", "\"gregrell/HW1\"", "false", "{\"login\":\"gregrell\",\"id\":16449334,\"node_id\":\"MDQ6VXNlcjE2NDQ5MzM0\",\"avatar_url\":\"https://avatars2.githubusercontent.com/u/16449334?v=4\",\"gravatar_id\":\"\",\"url\":\"https://api.github.com/users/gregrell\",\"html_url\":\"https://github.com/gregrell\",\"followers_url\":\"https://api.github.com/users/gregrell/followers\",\"following_url\":\"https://api.github.com/users/gregrell/following{/other_user}\",\"gists_url\":\"https://api.github.com/users/gregrell/gists{/gist_id}\",\"starred_url\":\"https://api.github.com/users/gregrell/starred{/owner}{/repo}\",\"subscriptions_url\":\"https://api.github.com/users/gregrell/subscriptions\",\"organizations_url\":\"https://api.github.com/users/gregrell/orgs\",\"repos_url\":\"https://api.github.com/users/gregrell/repos\",\"events_url\":\"https://api.github.com/users/gregrell/events{/privacy}\",\"received_events_url\":\"https://api.github.com/users/gregrell/received_events\",\"type\":\"User\",\"site_admin\":false}", "\"https://github.com/gregrell/HW1\"", "\"Grad school fall 2019 HW1. Not listing the course name so people in class can't grab my code\"", "false", "\"https://api.github.com/repos/gregrell/HW1\"", "\"https://api.github.com/repos/gregrell/HW1/forks\"", "\"https://api.github.com/repos/gregrell/HW1/keys{/key_id}\"", "\"https://api.github.com/repos/gregrell/HW1/collaborators{/collaborator}\"", "\"https://api.github.com/repos/gregrell/HW1/teams\"", "\"https://api.github.com/repos/gregrell/HW1/hooks\"", "\"https://api.github.com/repos/gregrell/HW1/issues/events{/number}\"", "\"https://api.github.com/repos/gregrell/HW1/events\"", "\"https://api.github.com/repos/gregrell/HW1/assignees{/user}\"", "\"https://api.github.com/repos/gregrell/HW1/branches{/branch}\"", "\"https://api.github.com/repos/gregrell/HW1/tags\"", "\"https://api.github.com/repos/gregrell/HW1/git/blobs{/sha}\"", "\"https://api.github.com/repos/gregrell/HW1/git/tags{/sha}\"", "\"https://api.github.com/repos/gregrell/HW1/git/refs{/sha}\"", "\"https://api.github.com/repos/gregrell/HW1/git/trees{/sha}\"", "\"https://api.github.com/repos/gregrell/HW1/statuses/{sha}\"", "\"https://api.github.com/repos/gregrell/HW1/languages\"", "\"https://api.github.com/repos/gregrell/HW1/stargazers\"", "\"https://api.github.com/repos/gregrell/HW1/contributors\"", "\"https://api.github.com/repos/gregrell/HW1/subscribers\"", "\"https://api.github.com/repos/gregrell/HW1/subscription\"", "\"https://api.github.com/repos/gregrell/HW1/commits{/sha}\"", "\"https://api.github.com/repos/gregrell/HW1/git/commits{/sha}\"", "\"https://api.github.com/repos/gregrell/HW1/comments{/number}\"", "\"https://api.github.com/repos/gregrell/HW1/issues/comments{/number}\"", "\"https://api.github.com/repos/gregrell/HW1/contents/{+path}\"", "\"https://api.github.com/repos/gregrell/HW1/compare/{base}...{head}\"", "\"https://api.github.com/repos/gregrell/HW1/merges\"", "\"https://api.github.com/repos/gregrell/HW1/{archive_format}{/ref}\"", "\"https://api.github.com/repos/gregrell/HW1/downloads\"", "\"https://api.github.com/repos/gregrell/HW1/issues{/number}\"", "\"https://api.github.com/repos/gregrell/HW1/pulls{/number}\"", "\"https://api.github.com/repos/gregrell/HW1/milestones{/number}\"", "\"https://api.github.com/repos/gregrell/HW1/notifications{?since,all,participating}\"", "\"https://api.github.com/repos/gregrell/HW1/labels{/name}\"", "\"https://api.github.com/repos/gregrell/HW1/releases{/id}\"", "\"https://api.github.com/repos/gregrell/HW1/deployments\"", "\"2019-09-13T13:32:51Z\"", "\"2019-09-19T21:05:34Z\"", "\"2019-09-19T21:05:32Z\"", "\"git://github.com/gregrell/HW1.git\"", "\"git@github.com:gregrell/HW1.git\"", "\"https://github.com/gregrell/HW1.git\"", "\"https://github.com/gregrell/HW1\"", "null", "2004", "0", "0", "\"Python\"", "true", "true", "true", "true", "false", "0", "null", "false", "false", "0", "null", "0", "0", "0", "\"master\""]], [["id", "node_id", "name", "full_name", "private", "owner", "html_url", "description", "fork", "url", "forks_url", "keys_url", "collaborators_url", "teams_url", "hooks_url", "issue_events_url", "events_url", "assignees_url", "branches_url", "tags_url", "blobs_url", "git_tags_url", "git_refs_url", "trees_url", "statuses_url", "languages_url", "stargazers_url", "contributors_url", "subscribers_url", "subscription_url", "commits_url", "git_commits_url", "comments_url", "issue_comment_url", "contents_url", "compare_url", "merges_url", "archive_url", "downloads_url", "issues_url", "pulls_url", "milestones_url", "notifications_url", "labels_url", "releases_url", "deployments_url", "created_at", "updated_at", "pushed_at", "git_url", "ssh_url", "clone_url", "svn_url", "homepage", "size", "stargazers_count", "watchers_count", "language", "has_issues", "has_projects", "has_downloads", "has_wiki", "has_pages", "forks_count", "mirror_url", "archived", "disabled", "open_issues_count", "license", "forks", "open_issues", "watchers", "default_branch"], ["213041097", "\"MDEwOlJlcG9zaXRvcnkyMTMwNDEwOTc=\"", "\"HW2\"", "\"gregrell/HW2\"", "false", "{\"login\":\"gregrell\",\"id\":16449334,\"node_id\":\"MDQ6VXNlcjE2NDQ5MzM0\",\"avatar_url\":\"https://avatars2.githubusercontent.com/u/16449334?v=4\",\"gravatar_id\":\"\",\"url\":\"https://api.github.com/users/gregrell\",\"html_url\":\"https://github.com/gregrell\",\"followers_url\":\"https://api.github.com/users/gregrell/followers\",\"following_url\":\"https://api.github.com/users/gregrell/following{/other_user}\",\"gists_url\":\"https://api.github.com/users/gregrell/gists{/gist_id}\",\"starred_url\":\"https://api.github.com/users/gregrell/starred{/owner}{/repo}\",\"subscriptions_url\":\"https://api.github.com/users/gregrell/subscriptions\",\"organizations_url\":\"https://api.github.com/users/gregrell/orgs\",\"repos_url\":\"https://api.github.com/users/gregrell/repos\",\"events_url\":\"https://api.github.com/users/gregrell/events{/privacy}\",\"received_events_url\":\"https://api.github.com/users/gregrell/received_events\",\"type\":\"User\",\"site_admin\":false}", "\"https://github.com/gregrell/HW2\"", "\"Text Classifier\"", "false", "\"https://api.github.com/repos/gregrell/HW2\"", "\"https://api.github.com/repos/gregrell/HW2/forks\"", "\"https://api.github.com/repos/gregrell/HW2/keys{/key_id}\"", "\"https://api.github.com/repos/gregrell/HW2/collaborators{/collaborator}\"", "\"https://api.github.com/repos/gregrell/HW2/teams\"", "\"https://api.github.com/repos/gregrell/HW2/hooks\"", "\"https://api.github.com/repos/gregrell/HW2/issues/events{/number}\"", "\"https://api.github.com/repos/gregrell/HW2/events\"", "\"https://api.github.com/repos/gregrell/HW2/assignees{/user}\"", "\"https://api.github.com/repos/gregrell/HW2/branches{/branch}\"", "\"https://api.github.com/repos/gregrell/HW2/tags\"", "\"https://api.github.com/repos/gregrell/HW2/git/blobs{/sha}\"", "\"https://api.github.com/repos/gregrell/HW2/git/tags{/sha}\"", "\"https://api.github.com/repos/gregrell/HW2/git/refs{/sha}\"", "\"https://api.github.com/repos/gregrell/HW2/git/trees{/sha}\"", "\"https://api.github.com/repos/gregrell/HW2/statuses/{sha}\"", "\"https://api.github.com/repos/gregrell/HW2/languages\"", "\"https://api.github.com/repos/gregrell/HW2/stargazers\"", "\"https://api.github.com/repos/gregrell/HW2/contributors\"", "\"https://api.github.com/repos/gregrell/HW2/subscribers\"", "\"https://api.github.com/repos/gregrell/HW2/subscription\"", "\"https://api.github.com/repos/gregrell/HW2/commits{/sha}\"", "\"https://api.github.com/repos/gregrell/HW2/git/commits{/sha}\"", "\"https://api.github.com/repos/gregrell/HW2/comments{/number}\"", "\"https://api.github.com/repos/gregrell/HW2/issues/comments{/number}\"", "\"https://api.github.com/repos/gregrell/HW2/contents/{+path}\"", "\"https://api.github.com/repos/gregrell/HW2/compare/{base}...{head}\"", "\"https://api.github.com/repos/gregrell/HW2/merges\"", "\"https://api.github.com/repos/gregrell/HW2/{archive_format}{/ref}\"", "\"https://api.github.com/repos/gregrell/HW2/downloads\"", "\"https://api.github.com/repos/gregrell/HW2/issues{/number}\"", "\"https://api.github.com/repos/gregrell/HW2/pulls{/number}\"", "\"https://api.github.com/repos/gregrell/HW2/milestones{/number}\"", "\"https://api.github.com/repos/gregrell/HW2/notifications{?since,all,participating}\"", "\"https://api.github.com/repos/gregrell/HW2/labels{/name}\"", "\"https://api.github.com/repos/gregrell/HW2/releases{/id}\"", "\"https://api.github.com/repos/gregrell/HW2/deployments\"", "\"2019-10-05T17:23:29Z\"", "\"2019-10-10T17:00:28Z\"", "\"2019-10-10T17:00:27Z\"", "\"git://github.com/gregrell/HW2.git\"", "\"git@github.com:gregrell/HW2.git\"", "\"https://github.com/gregrell/HW2.git\"", "\"https://github.com/gregrell/HW2\"", "null", "4392", "0", "0", "\"Python\"", "true", "true", "true", "true", "false", "0", "null", "false", "false", "0", "null", "0", "0", "0", "\"master\""]], [["id", "node_id", "name", "full_name", "private", "owner", "html_url", "description", "fork", "url", "forks_url", "keys_url", "collaborators_url", "teams_url", "hooks_url", "issue_events_url", "events_url", "assignees_url", "branches_url", "tags_url", "blobs_url", "git_tags_url", "git_refs_url", "trees_url", "statuses_url", "languages_url", "stargazers_url", "contributors_url", "subscribers_url", "subscription_url", "commits_url", "git_commits_url", "comments_url", "issue_comment_url", "contents_url", "compare_url", "merges_url", "archive_url", "downloads_url", "issues_url", "pulls_url", "milestones_url", "notifications_url", "labels_url", "releases_url", "deployments_url", "created_at", "updated_at", "pushed_at", "git_url", "ssh_url", "clone_url", "svn_url", "homepage", "size", "stargazers_count", "watchers_count", "language", "has_issues", "has_projects", "has_downloads", "has_wiki", "has_pages", "forks_count", "mirror_url", "archived", "disabled", "open_issues_count", "license", "forks", "open_issues", "watchers", "default_branch"], ["218944090", "\"MDEwOlJlcG9zaXRvcnkyMTg5NDQwOTA=\"", "\"HW3\"", "\"gregrell/HW3\"", "false", "{\"login\":\"gregrell\",\"id\":16449334,\"node_id\":\"MDQ6VXNlcjE2NDQ5MzM0\",\"avatar_url\":\"https://avatars2.githubusercontent.com/u/16449334?v=4\",\"gravatar_id\":\"\",\"url\":\"https://api.github.com/users/gregrell\",\"html_url\":\"https://github.com/gregrell\",\"followers_url\":\"https://api.github.com/users/gregrell/followers\",\"following_url\":\"https://api.github.com/users/gregrell/following{/other_user}\",\"gists_url\":\"https://api.github.com/users/gregrell/gists{/gist_id}\",\"starred_url\":\"https://api.github.com/users/gregrell/starred{/owner}{/repo}\",\"subscriptions_url\":\"https://api.github.com/users/gregrell/subscriptions\",\"organizations_url\":\"https://api.github.com/users/gregrell/orgs\",\"repos_url\":\"https://api.github.com/users/gregrell/repos\",\"events_url\":\"https://api.github.com/users/gregrell/events{/privacy}\",\"received_events_url\":\"https://api.github.com/users/gregrell/received_events\",\"type\":\"User\",\"site_admin\":false}", "\"https://github.com/gregrell/HW3\"", "null", "false", "\"https://api.github.com/repos/gregrell/HW3\"", "\"https://api.github.com/repos/gregrell/HW3/forks\"", "\"https://api.github.com/repos/gregrell/HW3/keys{/key_id}\"", "\"https://api.github.com/repos/gregrell/HW3/collaborators{/collaborator}\"", "\"https://api.github.com/repos/gregrell/HW3/teams\"", "\"https://api.github.com/repos/gregrell/HW3/hooks\"", "\"https://api.github.com/repos/gregrell/HW3/issues/events{/number}\"", "\"https://api.github.com/repos/gregrell/HW3/events\"", "\"https://api.github.com/repos/gregrell/HW3/assignees{/user}\"", "\"https://api.github.com/repos/gregrell/HW3/branches{/branch}\"", "\"https://api.github.com/repos/gregrell/HW3/tags\"", "\"https://api.github.com/repos/gregrell/HW3/git/blobs{/sha}\"", "\"https://api.github.com/repos/gregrell/HW3/git/tags{/sha}\"", "\"https://api.github.com/repos/gregrell/HW3/git/refs{/sha}\"", "\"https://api.github.com/repos/gregrell/HW3/git/trees{/sha}\"", "\"https://api.github.com/repos/gregrell/HW3/statuses/{sha}\"", "\"https://api.github.com/repos/gregrell/HW3/languages\"", "\"https://api.github.com/repos/gregrell/HW3/stargazers\"", "\"https://api.github.com/repos/gregrell/HW3/contributors\"", "\"https://api.github.com/repos/gregrell/HW3/subscribers\"", "\"https://api.github.com/repos/gregrell/HW3/subscription\"", "\"https://api.github.com/repos/gregrell/HW3/commits{/sha}\"", "\"https://api.github.com/repos/gregrell/HW3/git/commits{/sha}\"", "\"https://api.github.com/repos/gregrell/HW3/comments{/number}\"", "\"https://api.github.com/repos/gregrell/HW3/issues/comments{/number}\"", "\"https://api.github.com/repos/gregrell/HW3/contents/{+path}\"", "\"https://api.github.com/repos/gregrell/HW3/compare/{base}...{head}\"", "\"https://api.github.com/repos/gregrell/HW3/merges\"", "\"https://api.github.com/repos/gregrell/HW3/{archive_format}{/ref}\"", "\"https://api.github.com/repos/gregrell/HW3/downloads\"", "\"https://api.github.com/repos/gregrell/HW3/issues{/number}\"", "\"https://api.github.com/repos/gregrell/HW3/pulls{/number}\"", "\"https://api.github.com/repos/gregrell/HW3/milestones{/number}\"", "\"https://api.github.com/repos/gregrell/HW3/notifications{?since,all,participating}\"", "\"https://api.github.com/repos/gregrell/HW3/labels{/name}\"", "\"https://api.github.com/repos/gregrell/HW3/releases{/id}\"", "\"https://api.github.com/repos/gregrell/HW3/deployments\"", "\"2019-11-01T08:21:43Z\"", "\"2019-11-03T03:32:39Z\"", "\"2019-11-03T03:32:37Z\"", "\"git://github.com/gregrell/HW3.git\"", "\"git@github.com:gregrell/HW3.git\"", "\"https://github.com/gregrell/HW3.git\"", "\"https://github.com/gregrell/HW3\"", "null", "948", "0", "0", "\"Python\"", "true", "true", "true", "true", "false", "0", "null", "false", "false", "0", "null", "0", "0", "0", "\"master\""]], [["id", "node_id", "name", "full_name", "private", "owner", "html_url", "description", "fork", "url", "forks_url", "keys_url", "collaborators_url", "teams_url", "hooks_url", "issue_events_url", "events_url", "assignees_url", "branches_url", "tags_url", "blobs_url", "git_tags_url", "git_refs_url", "trees_url", "statuses_url", "languages_url", "stargazers_url", "contributors_url", "subscribers_url", "subscription_url", "commits_url", "git_commits_url", "comments_url", "issue_comment_url", "contents_url", "compare_url", "merges_url", "archive_url", "downloads_url", "issues_url", "pulls_url", "milestones_url", "notifications_url", "labels_url", "releases_url", "deployments_url", "created_at", "updated_at", "pushed_at", "git_url", "ssh_url", "clone_url", "svn_url", "homepage", "size", "stargazers_count", "watchers_count", "language", "has_issues", "has_projects", "has_downloads", "has_wiki", "has_pages", "forks_count", "mirror_url", "archived", "disabled", "open_issues_count", "license", "forks", "open_issues", "watchers", "default_branch"], ["64334212", "\"MDEwOlJlcG9zaXRvcnk2NDMzNDIxMg==\"", "\"Relearn\"", "\"gregrell/Relearn\"", "false", "{\"login\":\"gregrell\",\"id\":16449334,\"node_id\":\"MDQ6VXNlcjE2NDQ5MzM0\",\"avatar_url\":\"https://avatars2.githubusercontent.com/u/16449334?v=4\",\"gravatar_id\":\"\",\"url\":\"https://api.github.com/users/gregrell\",\"html_url\":\"https://github.com/gregrell\",\"followers_url\":\"https://api.github.com/users/gregrell/followers\",\"following_url\":\"https://api.github.com/users/gregrell/following{/other_user}\",\"gists_url\":\"https://api.github.com/users/gregrell/gists{/gist_id}\",\"starred_url\":\"https://api.github.com/users/gregrell/starred{/owner}{/repo}\",\"subscriptions_url\":\"https://api.github.com/users/gregrell/subscriptions\",\"organizations_url\":\"https://api.github.com/users/gregrell/orgs\",\"repos_url\":\"https://api.github.com/users/gregrell/repos\",\"events_url\":\"https://api.github.com/users/gregrell/events{/privacy}\",\"received_events_url\":\"https://api.github.com/users/gregrell/received_events\",\"type\":\"User\",\"site_admin\":false}", "\"https://github.com/gregrell/Relearn\"", "\"My own relearning Java Repo\"", "false", "\"https://api.github.com/repos/gregrell/Relearn\"", "\"https://api.github.com/repos/gregrell/Relearn/forks\"", "\"https://api.github.com/repos/gregrell/Relearn/keys{/key_id}\"", "\"https://api.github.com/repos/gregrell/Relearn/collaborators{/collaborator}\"", "\"https://api.github.com/repos/gregrell/Relearn/teams\"", "\"https://api.github.com/repos/gregrell/Relearn/hooks\"", "\"https://api.github.com/repos/gregrell/Relearn/issues/events{/number}\"", "\"https://api.github.com/repos/gregrell/Relearn/events\"", "\"https://api.github.com/repos/gregrell/Relearn/assignees{/user}\"", "\"https://api.github.com/repos/gregrell/Relearn/branches{/branch}\"", "\"https://api.github.com/repos/gregrell/Relearn/tags\"", "\"https://api.github.com/repos/gregrell/Relearn/git/blobs{/sha}\"", "\"https://api.github.com/repos/gregrell/Relearn/git/tags{/sha}\"", "\"https://api.github.com/repos/gregrell/Relearn/git/refs{/sha}\"", "\"https://api.github.com/repos/gregrell/Relearn/git/trees{/sha}\"", "\"https://api.github.com/repos/gregrell/Relearn/statuses/{sha}\"", "\"https://api.github.com/repos/gregrell/Relearn/languages\"", "\"https://api.github.com/repos/gregrell/Relearn/stargazers\"", "\"https://api.github.com/repos/gregrell/Relearn/contributors\"", "\"https://api.github.com/repos/gregrell/Relearn/subscribers\"", "\"https://api.github.com/repos/gregrell/Relearn/subscription\"", "\"https://api.github.com/repos/gregrell/Relearn/commits{/sha}\"", "\"https://api.github.com/repos/gregrell/Relearn/git/commits{/sha}\"", "\"https://api.github.com/repos/gregrell/Relearn/comments{/number}\"", "\"https://api.github.com/repos/gregrell/Relearn/issues/comments{/number}\"", "\"https://api.github.com/repos/gregrell/Relearn/contents/{+path}\"", "\"https://api.github.com/repos/gregrell/Relearn/compare/{base}...{head}\"", "\"https://api.github.com/repos/gregrell/Relearn/merges\"", "\"https://api.github.com/repos/gregrell/Relearn/{archive_format}{/ref}\"", "\"https://api.github.com/repos/gregrell/Relearn/downloads\"", "\"https://api.github.com/repos/gregrell/Relearn/issues{/number}\"", "\"https://api.github.com/repos/gregrell/Relearn/pulls{/number}\"", "\"https://api.github.com/repos/gregrell/Relearn/milestones{/number}\"", "\"https://api.github.com/repos/gregrell/Relearn/notifications{?since,all,participating}\"", "\"https://api.github.com/repos/gregrell/Relearn/labels{/name}\"", "\"https://api.github.com/repos/gregrell/Relearn/releases{/id}\"", "\"https://api.github.com/repos/gregrell/Relearn/deployments\"", "\"2016-07-27T18:57:18Z\"", "\"2016-07-28T06:23:30Z\"", "\"2016-08-01T05:54:08Z\"", "\"git://github.com/gregrell/Relearn.git\"", "\"git@github.com:gregrell/Relearn.git\"", "\"https://github.com/gregrell/Relearn.git\"", "\"https://github.com/gregrell/Relearn\"", "null", "31", "0", "0", "\"Java\"", "true", "true", "true", "true", "false", "0", "null", "false", "false", "0", "null", "0", "0", "0", "\"master\""]], [["id", "node_id", "name", "full_name", "private", "owner", "html_url", "description", "fork", "url", "forks_url", "keys_url", "collaborators_url", "teams_url", "hooks_url", "issue_events_url", "events_url", "assignees_url", "branches_url", "tags_url", "blobs_url", "git_tags_url", "git_refs_url", "trees_url", "statuses_url", "languages_url", "stargazers_url", "contributors_url", "subscribers_url", "subscription_url", "commits_url", "git_commits_url", "comments_url", "issue_comment_url", "contents_url", "compare_url", "merges_url", "archive_url", "downloads_url", "issues_url", "pulls_url", "milestones_url", "notifications_url", "labels_url", "releases_url", "deployments_url", "created_at", "updated_at", "pushed_at", "git_url", "ssh_url", "clone_url", "svn_url", "homepage", "size", "stargazers_count", "watchers_count", "language", "has_issues", "has_projects", "has_downloads", "has_wiki", "has_pages", "forks_count", "mirror_url", "archived", "disabled", "open_issues_count", "license", "forks", "open_issues", "watchers", "default_branch"], ["214243415", "\"MDEwOlJlcG9zaXRvcnkyMTQyNDM0MTU=\"", "\"TestGen\"", "\"gregrell/TestGen\"", "false", "{\"login\":\"gregrell\",\"id\":16449334,\"node_id\":\"MDQ6VXNlcjE2NDQ5MzM0\",\"avatar_url\":\"https://avatars2.githubusercontent.com/u/16449334?v=4\",\"gravatar_id\":\"\",\"url\":\"https://api.github.com/users/gregrell\",\"html_url\":\"https://github.com/gregrell\",\"followers_url\":\"https://api.github.com/users/gregrell/followers\",\"following_url\":\"https://api.github.com/users/gregrell/following{/other_user}\",\"gists_url\":\"https://api.github.com/users/gregrell/gists{/gist_id}\",\"starred_url\":\"https://api.github.com/users/gregrell/starred{/owner}{/repo}\",\"subscriptions_url\":\"https://api.github.com/users/gregrell/subscriptions\",\"organizations_url\":\"https://api.github.com/users/gregrell/orgs\",\"repos_url\":\"https://api.github.com/users/gregrell/repos\",\"events_url\":\"https://api.github.com/users/gregrell/events{/privacy}\",\"received_events_url\":\"https://api.github.com/users/gregrell/received_events\",\"type\":\"User\",\"site_admin\":false}", "\"https://github.com/gregrell/TestGen\"", "\"Test Generator\"", "false", "\"https://api.github.com/repos/gregrell/TestGen\"", "\"https://api.github.com/repos/gregrell/TestGen/forks\"", "\"https://api.github.com/repos/gregrell/TestGen/keys{/key_id}\"", "\"https://api.github.com/repos/gregrell/TestGen/collaborators{/collaborator}\"", "\"https://api.github.com/repos/gregrell/TestGen/teams\"", "\"https://api.github.com/repos/gregrell/TestGen/hooks\"", "\"https://api.github.com/repos/gregrell/TestGen/issues/events{/number}\"", "\"https://api.github.com/repos/gregrell/TestGen/events\"", "\"https://api.github.com/repos/gregrell/TestGen/assignees{/user}\"", "\"https://api.github.com/repos/gregrell/TestGen/branches{/branch}\"", "\"https://api.github.com/repos/gregrell/TestGen/tags\"", "\"https://api.github.com/repos/gregrell/TestGen/git/blobs{/sha}\"", "\"https://api.github.com/repos/gregrell/TestGen/git/tags{/sha}\"", "\"https://api.github.com/repos/gregrell/TestGen/git/refs{/sha}\"", "\"https://api.github.com/repos/gregrell/TestGen/git/trees{/sha}\"", "\"https://api.github.com/repos/gregrell/TestGen/statuses/{sha}\"", "\"https://api.github.com/repos/gregrell/TestGen/languages\"", "\"https://api.github.com/repos/gregrell/TestGen/stargazers\"", "\"https://api.github.com/repos/gregrell/TestGen/contributors\"", "\"https://api.github.com/repos/gregrell/TestGen/subscribers\"", "\"https://api.github.com/repos/gregrell/TestGen/subscription\"", "\"https://api.github.com/repos/gregrell/TestGen/commits{/sha}\"", "\"https://api.github.com/repos/gregrell/TestGen/git/commits{/sha}\"", "\"https://api.github.com/repos/gregrell/TestGen/comments{/number}\"", "\"https://api.github.com/repos/gregrell/TestGen/issues/comments{/number}\"", "\"https://api.github.com/repos/gregrell/TestGen/contents/{+path}\"", "\"https://api.github.com/repos/gregrell/TestGen/compare/{base}...{head}\"", "\"https://api.github.com/repos/gregrell/TestGen/merges\"", "\"https://api.github.com/repos/gregrell/TestGen/{archive_format}{/ref}\"", "\"https://api.github.com/repos/gregrell/TestGen/downloads\"", "\"https://api.github.com/repos/gregrell/TestGen/issues{/number}\"", "\"https://api.github.com/repos/gregrell/TestGen/pulls{/number}\"", "\"https://api.github.com/repos/gregrell/TestGen/milestones{/number}\"", "\"https://api.github.com/repos/gregrell/TestGen/notifications{?since,all,participating}\"", "\"https://api.github.com/repos/gregrell/TestGen/labels{/name}\"", "\"https://api.github.com/repos/gregrell/TestGen/releases{/id}\"", "\"https://api.github.com/repos/gregrell/TestGen/deployments\"", "\"2019-10-10T17:22:50Z\"", "\"2019-10-23T21:12:31Z\"", "\"2019-10-23T21:12:29Z\"", "\"git://github.com/gregrell/TestGen.git\"", "\"git@github.com:gregrell/TestGen.git\"", "\"https://github.com/gregrell/TestGen.git\"", "\"https://github.com/gregrell/TestGen\"", "null", "12", "0", "0", "\"Python\"", "true", "true", "true", "true", "false", "0", "null", "false", "false", "0", "null", "0", "0", "0", "\"master\""]], [["id", "node_id", "name", "full_name", "private", "owner", "html_url", "description", "fork", "url", "forks_url", "keys_url", "collaborators_url", "teams_url", "hooks_url", "issue_events_url", "events_url", "assignees_url", "branches_url", "tags_url", "blobs_url", "git_tags_url", "git_refs_url", "trees_url", "statuses_url", "languages_url", "stargazers_url", "contributors_url", "subscribers_url", "subscription_url", "commits_url", "git_commits_url", "comments_url", "issue_comment_url", "contents_url", "compare_url", "merges_url", "archive_url", "downloads_url", "issues_url", "pulls_url", "milestones_url", "notifications_url", "labels_url", "releases_url", "deployments_url", "created_at", "updated_at", "pushed_at", "git_url", "ssh_url", "clone_url", "svn_url", "homepage", "size", "stargazers_count", "watchers_count", "language", "has_issues", "has_projects", "has_downloads", "has_wiki", "has_pages", "forks_count", "mirror_url", "archived", "disabled", "open_issues_count", "license", "forks", "open_issues", "watchers", "default_branch"], ["264550697", "\"MDEwOlJlcG9zaXRvcnkyNjQ1NTA2OTc=\"", "\"UCAS\"", "\"gregrell/UCAS\"", "false", "{\"login\":\"gregrell\",\"id\":16449334,\"node_id\":\"MDQ6VXNlcjE2NDQ5MzM0\",\"avatar_url\":\"https://avatars2.githubusercontent.com/u/16449334?v=4\",\"gravatar_id\":\"\",\"url\":\"https://api.github.com/users/gregrell\",\"html_url\":\"https://github.com/gregrell\",\"followers_url\":\"https://api.github.com/users/gregrell/followers\",\"following_url\":\"https://api.github.com/users/gregrell/following{/other_user}\",\"gists_url\":\"https://api.github.com/users/gregrell/gists{/gist_id}\",\"starred_url\":\"https://api.github.com/users/gregrell/starred{/owner}{/repo}\",\"subscriptions_url\":\"https://api.github.com/users/gregrell/subscriptions\",\"organizations_url\":\"https://api.github.com/users/gregrell/orgs\",\"repos_url\":\"https://api.github.com/users/gregrell/repos\",\"events_url\":\"https://api.github.com/users/gregrell/events{/privacy}\",\"received_events_url\":\"https://api.github.com/users/gregrell/received_events\",\"type\":\"User\",\"site_admin\":false}", "\"https://github.com/gregrell/UCAS\"", "null", "false", "\"https://api.github.com/repos/gregrell/UCAS\"", "\"https://api.github.com/repos/gregrell/UCAS/forks\"", "\"https://api.github.com/repos/gregrell/UCAS/keys{/key_id}\"", "\"https://api.github.com/repos/gregrell/UCAS/collaborators{/collaborator}\"", "\"https://api.github.com/repos/gregrell/UCAS/teams\"", "\"https://api.github.com/repos/gregrell/UCAS/hooks\"", "\"https://api.github.com/repos/gregrell/UCAS/issues/events{/number}\"", "\"https://api.github.com/repos/gregrell/UCAS/events\"", "\"https://api.github.com/repos/gregrell/UCAS/assignees{/user}\"", "\"https://api.github.com/repos/gregrell/UCAS/branches{/branch}\"", "\"https://api.github.com/repos/gregrell/UCAS/tags\"", "\"https://api.github.com/repos/gregrell/UCAS/git/blobs{/sha}\"", "\"https://api.github.com/repos/gregrell/UCAS/git/tags{/sha}\"", "\"https://api.github.com/repos/gregrell/UCAS/git/refs{/sha}\"", "\"https://api.github.com/repos/gregrell/UCAS/git/trees{/sha}\"", "\"https://api.github.com/repos/gregrell/UCAS/statuses/{sha}\"", "\"https://api.github.com/repos/gregrell/UCAS/languages\"", "\"https://api.github.com/repos/gregrell/UCAS/stargazers\"", "\"https://api.github.com/repos/gregrell/UCAS/contributors\"", "\"https://api.github.com/repos/gregrell/UCAS/subscribers\"", "\"https://api.github.com/repos/gregrell/UCAS/subscription\"", "\"https://api.github.com/repos/gregrell/UCAS/commits{/sha}\"", "\"https://api.github.com/repos/gregrell/UCAS/git/commits{/sha}\"", "\"https://api.github.com/repos/gregrell/UCAS/comments{/number}\"", "\"https://api.github.com/repos/gregrell/UCAS/issues/comments{/number}\"", "\"https://api.github.com/repos/gregrell/UCAS/contents/{+path}\"", "\"https://api.github.com/repos/gregrell/UCAS/compare/{base}...{head}\"", "\"https://api.github.com/repos/gregrell/UCAS/merges\"", "\"https://api.github.com/repos/gregrell/UCAS/{archive_format}{/ref}\"", "\"https://api.github.com/repos/gregrell/UCAS/downloads\"", "\"https://api.github.com/repos/gregrell/UCAS/issues{/number}\"", "\"https://api.github.com/repos/gregrell/UCAS/pulls{/number}\"", "\"https://api.github.com/repos/gregrell/UCAS/milestones{/number}\"", "\"https://api.github.com/repos/gregrell/UCAS/notifications{?since,all,participating}\"", "\"https://api.github.com/repos/gregrell/UCAS/labels{/name}\"", "\"https://api.github.com/repos/gregrell/UCAS/releases{/id}\"", "\"https://api.github.com/repos/gregrell/UCAS/deployments\"", "\"2020-05-17T00:01:17Z\"", "\"2020-06-15T08:21:08Z\"", "\"2020-06-15T08:21:05Z\"", "\"git://github.com/gregrell/UCAS.git\"", "\"git@github.com:gregrell/UCAS.git\"", "\"https://github.com/gregrell/UCAS.git\"", "\"https://github.com/gregrell/UCAS\"", "null", "7537", "0", "0", "\"LabVIEW\"", "true", "true", "true", "true", "false", "0", "null", "false", "false", "0", "null", "0", "0", "0", "\"master\""]], [["id", "node_id", "name", "full_name", "private", "owner", "html_url", "description", "fork", "url", "forks_url", "keys_url", "collaborators_url", "teams_url", "hooks_url", "issue_events_url", "events_url", "assignees_url", "branches_url", "tags_url", "blobs_url", "git_tags_url", "git_refs_url", "trees_url", "statuses_url", "languages_url", "stargazers_url", "contributors_url", "subscribers_url", "subscription_url", "commits_url", "git_commits_url", "comments_url", "issue_comment_url", "contents_url", "compare_url", "merges_url", "archive_url", "downloads_url", "issues_url", "pulls_url", "milestones_url", "notifications_url", "labels_url", "releases_url", "deployments_url", "created_at", "updated_at", "pushed_at", "git_url", "ssh_url", "clone_url", "svn_url", "homepage", "size", "stargazers_count", "watchers_count", "language", "has_issues", "has_projects", "has_downloads", "has_wiki", "has_pages", "forks_count", "mirror_url", "archived", "disabled", "open_issues_count", "license", "forks", "open_issues", "watchers", "default_branch"], ["261532152", "\"MDEwOlJlcG9zaXRvcnkyNjE1MzIxNTI=\"", "\"VisualMac\"", "\"gregrell/VisualMac\"", "false", "{\"login\":\"gregrell\",\"id\":16449334,\"node_id\":\"MDQ6VXNlcjE2NDQ5MzM0\",\"avatar_url\":\"https://avatars2.githubusercontent.com/u/16449334?v=4\",\"gravatar_id\":\"\",\"url\":\"https://api.github.com/users/gregrell\",\"html_url\":\"https://github.com/gregrell\",\"followers_url\":\"https://api.github.com/users/gregrell/followers\",\"following_url\":\"https://api.github.com/users/gregrell/following{/other_user}\",\"gists_url\":\"https://api.github.com/users/gregrell/gists{/gist_id}\",\"starred_url\":\"https://api.github.com/users/gregrell/starred{/owner}{/repo}\",\"subscriptions_url\":\"https://api.github.com/users/gregrell/subscriptions\",\"organizations_url\":\"https://api.github.com/users/gregrell/orgs\",\"repos_url\":\"https://api.github.com/users/gregrell/repos\",\"events_url\":\"https://api.github.com/users/gregrell/events{/privacy}\",\"received_events_url\":\"https://api.github.com/users/gregrell/received_events\",\"type\":\"User\",\"site_admin\":false}", "\"https://github.com/gregrell/VisualMac\"", "\"getting acquainted with the hell that is Mac and C#\"", "false", "\"https://api.github.com/repos/gregrell/VisualMac\"", "\"https://api.github.com/repos/gregrell/VisualMac/forks\"", "\"https://api.github.com/repos/gregrell/VisualMac/keys{/key_id}\"", "\"https://api.github.com/repos/gregrell/VisualMac/collaborators{/collaborator}\"", "\"https://api.github.com/repos/gregrell/VisualMac/teams\"", "\"https://api.github.com/repos/gregrell/VisualMac/hooks\"", "\"https://api.github.com/repos/gregrell/VisualMac/issues/events{/number}\"", "\"https://api.github.com/repos/gregrell/VisualMac/events\"", "\"https://api.github.com/repos/gregrell/VisualMac/assignees{/user}\"", "\"https://api.github.com/repos/gregrell/VisualMac/branches{/branch}\"", "\"https://api.github.com/repos/gregrell/VisualMac/tags\"", "\"https://api.github.com/repos/gregrell/VisualMac/git/blobs{/sha}\"", "\"https://api.github.com/repos/gregrell/VisualMac/git/tags{/sha}\"", "\"https://api.github.com/repos/gregrell/VisualMac/git/refs{/sha}\"", "\"https://api.github.com/repos/gregrell/VisualMac/git/trees{/sha}\"", "\"https://api.github.com/repos/gregrell/VisualMac/statuses/{sha}\"", "\"https://api.github.com/repos/gregrell/VisualMac/languages\"", "\"https://api.github.com/repos/gregrell/VisualMac/stargazers\"", "\"https://api.github.com/repos/gregrell/VisualMac/contributors\"", "\"https://api.github.com/repos/gregrell/VisualMac/subscribers\"", "\"https://api.github.com/repos/gregrell/VisualMac/subscription\"", "\"https://api.github.com/repos/gregrell/VisualMac/commits{/sha}\"", "\"https://api.github.com/repos/gregrell/VisualMac/git/commits{/sha}\"", "\"https://api.github.com/repos/gregrell/VisualMac/comments{/number}\"", "\"https://api.github.com/repos/gregrell/VisualMac/issues/comments{/number}\"", "\"https://api.github.com/repos/gregrell/VisualMac/contents/{+path}\"", "\"https://api.github.com/repos/gregrell/VisualMac/compare/{base}...{head}\"", "\"https://api.github.com/repos/gregrell/VisualMac/merges\"", "\"https://api.github.com/repos/gregrell/VisualMac/{archive_format}{/ref}\"", "\"https://api.github.com/repos/gregrell/VisualMac/downloads\"", "\"https://api.github.com/repos/gregrell/VisualMac/issues{/number}\"", "\"https://api.github.com/repos/gregrell/VisualMac/pulls{/number}\"", "\"https://api.github.com/repos/gregrell/VisualMac/milestones{/number}\"", "\"https://api.github.com/repos/gregrell/VisualMac/notifications{?since,all,participating}\"", "\"https://api.github.com/repos/gregrell/VisualMac/labels{/name}\"", "\"https://api.github.com/repos/gregrell/VisualMac/releases{/id}\"", "\"https://api.github.com/repos/gregrell/VisualMac/deployments\"", "\"2020-05-05T16:56:06Z\"", "\"2020-05-11T16:12:31Z\"", "\"2020-05-11T16:12:29Z\"", "\"git://github.com/gregrell/VisualMac.git\"", "\"git@github.com:gregrell/VisualMac.git\"", "\"https://github.com/gregrell/VisualMac.git\"", "\"https://github.com/gregrell/VisualMac\"", "null", "277", "0", "0", "\"C#\"", "true", "true", "true", "true", "false", "0", "null", "false", "false", "0", "null", "0", "0", "0", "\"master\""]]]
  # "\"https://api.github.com/repos/gregrell/6135-A1\""
  # "\"https://api.github.com/repos/gregrell/6135-A1/git/commits{/sha}\""
  n1 = call <vilib>:"Create REST Client.vi"("Verify Server(true)"=FALSE, "Authentication"=cluster{"Username":string, "Password":string} {"Username"="rell.greg@gmail.com", "Password"="qpmzgh740!!"}, "Escape URLs (true)"=TRUE, "Base URL"="") -> ("error out"=w9:errorcluster, "REST Client out"=w12:refnum<class "REST Client.lvclass">)  [unwired: 6 in]
  n2 = call-dynamic "HTTP GET.vi"("error in (no error)"=w9, "Path"="https://api.github.com/users/gregrell/repos", "REST Client in"=w12) -> ("error out"=w5:errorcluster, "Response body"=w6:string)  [unwired: 3 in, 4 out]
  n3 = call <vilib>:"Get Array Elements.vi"("error in (no error)"=w5, "JSON"=w6) -> ("error out"=w4:errorcluster, "<JSON>"=w3:string[])  [unwired: 7 in, 1 out]
  n4 = case shown="No Error" w4 {
    tunnel: w3 -> [w15 _]
    tunnel: [w14 string[][][] []] -> w2
    frame No Error {
      n5 = for {
        tunnel: w15 -> [w19] mode=indexing
        tunnel: [w16] -> w14 mode=indexing
        n6 = call <vilib>:"Get all Object Items.vi"("JSON"=w19) -> ("<JSON>"=w17:string[], "Item Names"=w18:string[])  [unwired: 7 in, 2 out]
        n7 = Build Array(w18, w17) -> (w16:string[][])
      }
    }
    frame Error {
    }
  }
  n8 = for {
    tunnel: w2 -> [w31] mode=indexing
    tunnel: [w42] -> w1 mode=indexing
    n9 = call "Git-Get Repo Info by Key.vi"("Repo Info"=w31, "Key"="id" ("element")) -> ("<JSON>"=w43:string)  [unwired: 9 in]
    n10 = call "Git-Get Repo Info by Key.vi"("Repo Info"=w31, "Key"="node_id" ("element")) -> ("<JSON>"=w30:string)  [unwired: 9 in]
    n11 = call "Git-Get Repo Info by Key.vi"("Repo Info"=w31, "Key"="name" ("element")) -> ("<JSON>"=w29:string)  [unwired: 9 in]
    n12 = call "Git-Get Repo Info by Key.vi"("Repo Info"=w31, "Key"="full_name" ("element")) -> ("<JSON>"=w28:string)  [unwired: 9 in]
    n13 = call "Git-Get Repo Info by Key.vi"("Repo Info"=w31, "Key"="private" ("element")) -> ("<JSON>"=w27:string)  [unwired: 9 in]
    n14 = call "Git-Get Repo Info by Key.vi"("Repo Info"=w31, "Key"="owner" ("element")) -> ("<JSON>"=w26:string)  [unwired: 9 in]
    n15 = call "Git-Get Repo Info by Key.vi"("Repo Info"=w31, "Key"="html_url" ("element")) -> ("<JSON>"=w25:string)  [unwired: 9 in]
    n16 = call "Git-Get Repo Info by Key.vi"("Repo Info"=w31, "Key"="description" ("element")) -> ("<JSON>"=w24:string)  [unwired: 9 in]
    n17 = call "Git-Get Repo Info by Key.vi"("Repo Info"=w31, "Key"="url" ("element")) -> ("<JSON>"=w23:string)  [unwired: 9 in]
    n18 = call "Git-Get Repo Info by Key.vi"("Repo Info"=w31, "Key"="collaborators_url" ("element")) -> ("<JSON>"=w22:string)  [unwired: 9 in]
    n19 = call "Git-Get Repo Info by Key.vi"("Repo Info"=w31, "Key"="teams_url" ("element")) -> ("<JSON>"=w21:string)  [unwired: 9 in]
    n20 = Bundle By Name(cluster=T1 {"ID"="", "node_id"="", "name"="", "full_name"="", "private"="", "owner"="", "html_url"="", "description"="", "url"="", "collaborators_url"="", "teams_url"=""}, "ID"=w43, "node_id"=w30, "name"=w29, "full_name"=w28, "private"=w27, "owner"=w26, "html_url"=w25, "description"=w24, "url"=w23, "collaborators_url"=w22, "teams_url"=w21) -> (w42:T1)
  }
  "Array" <- w1
